vi "Get DAQData Dict.vi"(8 "error in (no error)":errorcluster, 11 "DAQ":refnum<class "DAQ.lvclass">) -> (0 "error out":errorcluster, 2 "DAQ Data Dict DVR":T1, 3 "DAQ":refnum<class "DAQ.lvclass">)   [LabVIEW 2017, in "DAQ.lvclass"]
doc: "Developed by Kevin Thompson\nkevin@thompsonengineering.net\n\nCopyright 2018-2020\nThompson Engineering, LLC"
uses:
  DAQ.lvclass
  <vilib>/TELLC/Dynamic CVT API/TD Dynamic CVT DVR--ref.ctl
  DAQ.lvclass/DAQ.ctl
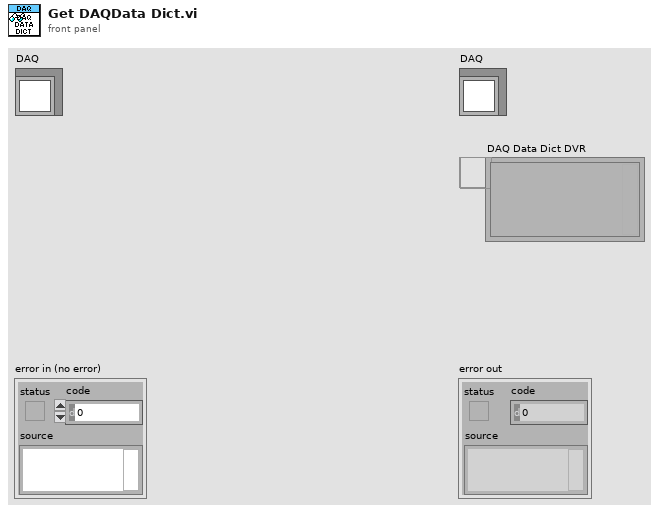
[diagram p1: front panel]
types:
  T1 = typedef "TD Dynamic CVT DVR--ref.ctl" = refnum<data-value>
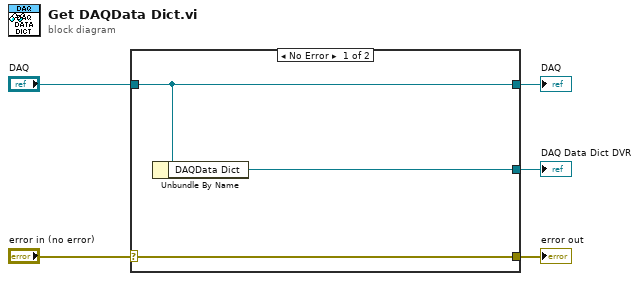
[diagram p0: block diagram]
diagram:
  n1 = case shown="No Error" "error in (no error)" {
    selector: "error in (no error)" -> [w8 w9]
    tunnel: [w8 w9] -> w4
    tunnel: [w7 w10] -> w2
    tunnel: "DAQ" -> [w7 w10]
    tunnel: [w6 _] -> w1
    frame No Error {
      n2 = Unbundle By Name(w7) -> ("DAQData Dict"=w6:T1)
    }
    frame Error {
    }
  }
  "error out" <- w4
  "DAQ" <- w2
  "DAQ Data Dict DVR" <- w1
